vi "SelectTag.vi"(11 "Tag in":T1) -> (2 "Canceled?":bool, 3 "Tag out":T1)   [LabVIEW 2016, in "Systemlink Tag.xctl"]
uses:
  <userlib>/MicroPython/VIs/SystemLink/Systemlink Tag.xctl
  <userlib>/MicroPython/VIs/SystemLink/Systemlink Data.ctl
panel:
  in  "IO":cluster{"Cancel Button":bool, "OK Button":bool}
  in  "Delete Tag":bool
  in  "Refresh Button":bool
  in  "New Tag":bool
  in  "Tags":i32(listbox)=-1
  # "SystemLink Panel\n\nhttps://www.systemlinkcloud.com\n\nAPI: https://api.systemlinkcloud.com"
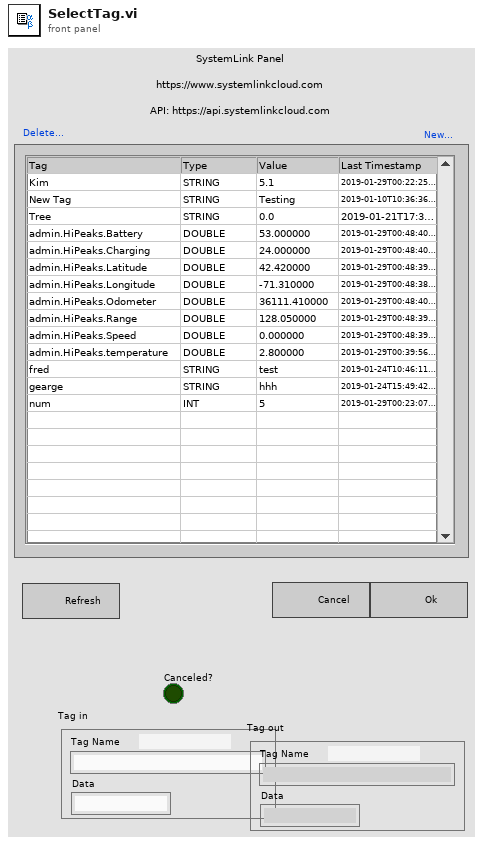
[diagram p1: front panel]
types:
  T1 = typedef "Systemlink Tag.xctl/Systemlink Data.ctl" = cluster{"Tag Name":string, "Type":string, "Data":string}
  T2 = enum8{"Enabled", "Disabled", "Disabled and Grayed Out"}
  T3 = typedef "SkylineCluster.ctl" = cluster{"Name":string, "BaseURL":string, "AppKey":string, "Headers":string[], "Timeout":i32}
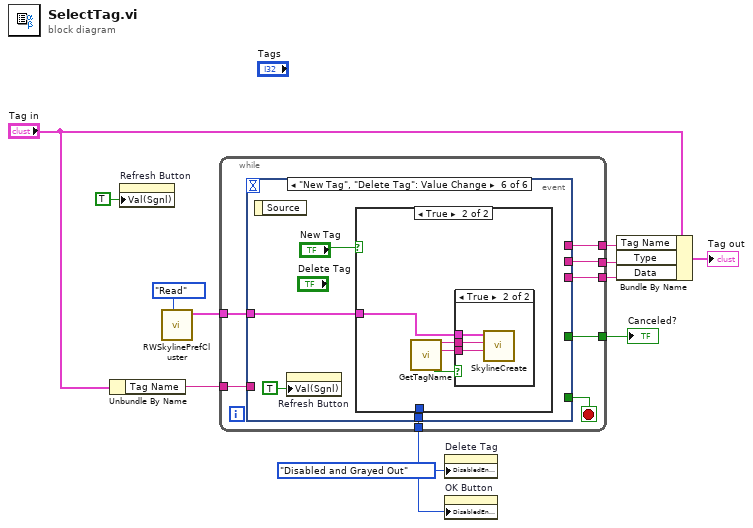
[diagram p0: block diagram]
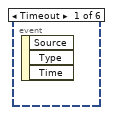
[diagram p2: hidden frame]
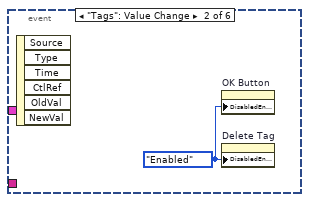
[diagram p3: hidden frame]
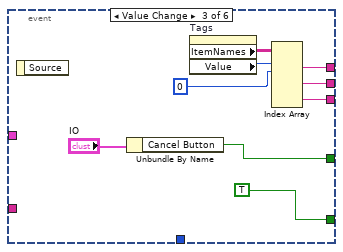
[diagram p4: hidden frame]
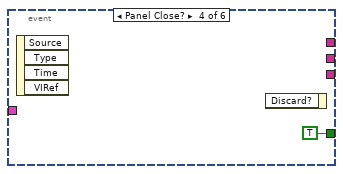
[diagram p5: hidden frame]
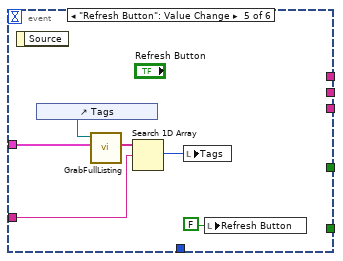
[diagram p6: hidden frame]
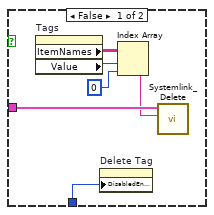
[diagram p7: hidden frame]
diagram:
  w1 = T2."Disabled and Grayed Out" ("Disabled")
  n1 = Unbundle By Name("Tag in") -> ("Tag Name"=w4:string)
  n2 = property on="Refresh Button" class="Bool (strict)"("Val(Sgnl)"=TRUE ("Value (Signaling)")) -> ()  [unwired: 2 in, 2 out]
  n3 = call <userlib>:"RWSkylinePrefCluster.vi"("Task"=enum16{"Read", "Write"}."Read") -> ("Device Out"=w3:T3)  [unwired: 9 in, 1 out]
  n4 = while {
    tunnel: [w18] -> w9
    tunnel: [w17] -> w11
    tunnel: [w16] -> w8
    tunnel: [w15] -> w7
    tunnel: w3 -> [w14]
    tunnel: w4 -> [w13]
    tunnel: w1 -> [w12]
    stop <- w19 stop-if-true
    n5 = event shown="[5] \"New Tag\", \"Delete Tag\": Value Change" {
      selector: _ -> [_ _ _ _ _ _]
      dyn-events: _ -> [_ _ _ _ _ _]
      timeout: _ -> [_ _ _ _ _ _]
      tunnel: [_ _ TRUE _ _ _] -> w19
      tunnel: [_ _ w25 _ _ _] -> w18
      tunnel: [_ _ w21 TRUE ("Cancel Button") _ _] -> w17
      tunnel: [_ _ w24 _ _ _] -> w16
      tunnel: [_ _ w23 _ _ _] -> w15
      tunnel: w14 -> [_ _ _ _ w36 w38]
      tunnel: w13 -> [_ _ _ _ w32 _]
      tunnel: w12 -> [_ _ _ _ _ w37]
      event Timeout {
        n6 = event-data() -> ()  [unwired: 1 in, 3 out]
      }
      event "Tags": Value Change {
        w20 = T2."Enabled" ("Disabled")
        n7 = event-data() -> ()  [unwired: 1 in, 6 out]
        n8 = property on="OK Button" class="Bool"("DisabledEnum"=w20) -> ()  [unwired: 2 in, 2 out]
        n9 = property on="Delete Tag" class="Bool"("DisabledEnum"=w20) -> ()  [unwired: 2 in, 2 out]
      }
      event "IO.OK Button", "IO.Cancel Button": Value Change {
        n10 = event-data() -> ()  [unwired: 1 in, 1 out]
        n11 = Unbundle By Name("IO") -> ("Cancel Button"=w21:bool)
        n12 = property on="Tags" class="MCListbox (strict)"() -> ("ItemNames"=w29:string[][], "Value"=w28:i32)  [unwired: 2 in, 2 out]
        n13 = Index Array(array=w29, index (row) #1=w28, index (col) #1=0 ("disabled index (col)")) -> (element #1=w25:string, element #2=w24:string, element #3=w23:string)  [unwired: 4 in]
      }
      event Panel Close? {
        n14 = event-data() -> ()  [unwired: 1 in, 4 out]
        n15 = event-data() -> ()  [unwired: 2 in, 1 out]
      }
      event "Refresh Button": Value Change {
        n16 = event-data() -> ()  [unwired: 1 in, 1 out]
        n17 = control-ref of="Tags"() -> (w35:refnum<vi>)
        n18 = call <userlib>:"GrabFullListing.vi"("Device In"=w36, "MulticolumnListbox in"=w35) -> ("tags"=w33:string[])  [unwired: 9 in]
        n19 = Search 1D Array(1D array=w33, element=w32) -> (index of element=w31:i32)  [unwired: 1 in]
        n20 = local write "Tags"(w31) -> ()
        n21 = local write "Refresh Button"(FALSE ("Refresh Button")) -> ()
      }
      event "New Tag", "Delete Tag": Value Change {
        n22 = event-data() -> ()  [unwired: 1 in, 1 out]
        n23 = property on="Refresh Button" class="Bool (strict)"("Val(Sgnl)"=TRUE ("Value (Signaling)")) -> ()  [unwired: 2 in, 2 out]
        n24 = case shown="True" "New Tag" {
          tunnel: w38 -> [w46 w50]
          tunnel: w37 -> [w41 _]
          frame False {
            n25 = property on="Tags" class="MCListbox (strict)"() -> ("ItemNames"=w45:string[][], "Value"=w44:i32)  [unwired: 2 in, 2 out]
            n26 = property on="Delete Tag" class="Bool"("DisabledEnum"=w41) -> ()  [unwired: 2 in, 2 out]
            n27 = Index Array(array=w45, index (row)=w44, index (col)=0 ("disabled index (col)")) -> (element=w42:string)
            n28 = call <userlib>:"Systemlink_Delete.vi"("Tag Path"=w42, "Device In"=w46) -> ()  [unwired: 10 in]
          }
          frame True {
            n29 = call <userlib>:"GetTagName.vi"() -> ("OK"=w47:bool, "Type"=w48:string, "Name"=w49:string)  [unwired: 3 in]
            n30 = case shown="True" w47 {
              tunnel: w50 -> [_ w53]
              tunnel: w49 -> [_ w52]
              tunnel: w48 -> [_ w51]
              frame False {
              }
              frame True {
                n31 = call <userlib>:"SkylineCreate.vi"("Type"=w51, "tag"=w52, "Device In"=w53) -> ()  [unwired: 6 in, 3 out]
              }
            }
          }
        }
      }
    }
  }
  "Canceled?" <- w11
  n32 = property on="Delete Tag" class="Bool"("DisabledEnum"=w1) -> ()  [unwired: 2 in, 2 out]
  n33 = property on="OK Button" class="Bool"("DisabledEnum"=w1) -> ()  [unwired: 2 in, 2 out]
  n34 = Bundle By Name(cluster="Tag in", "Tag Name"=w9, "Type"=w8, "Data"=w7) -> (→"Tag out":T1)
